vi "CAN Communication.vi"() -> ()   [LabVIEW 2011]
uses:
  <vilib>/Analysis/NI_AALBase.lvlib
panel:
  out "flag":bool
  out "Bias":dbl[](array[numeric]) format="%#.0f"
  out "ForceTorque":dbl[](array[numeric])
  in  "Overall TAP":enum32{"Graph", "CAN Activate"}(tab)
  in  "UNBIAS(SW)":bool
  in  "Control Box":T1={"Rotate & Translate"=FALSE, "rotation angle"=0.0, "Force Divider"=50.0, "Torque Divider"=2000.0}
  in  "BIAS(SW)":bool
  out "Tz":dbl(graph)
  out "Ty":dbl(graph)
  out "Tx":dbl(graph)
  out "Fz":dbl(graph)
  out "Fy":dbl(graph)
  out "Fx":dbl(graph)
  in  "Stop":bool
  in  "FT 출력":bool
  in  "Command":bool
  in  "Command":u16(ring)=11 items=["Not yet - Read Model Name", "Not yet - Read S/N", "Not yet - Read Firmware Ver.", "Set Communication ID", "Not yet - Read Communication ID", "UART version only - Set Baud-rate", "UART version only - Read Baud-rate", "Set Filter", "Not yet - Read Filter Setting", "F/T 1 sample Output", "F/T Output", "F/T Output Stop", "Reserved", "Reserved", "Set Output Rate", "Not yet -Read Output Rate", "Not yet -Bias Setting", "Not yet -Read Overload log"]
  in  "Set 2":T2={"Filter Type"=0, "Baud-rate"=0, "Output Rate"=0, "Cutoff Frequency"=0, "Receiving ID"=100, "Transmitting ID First "=1, "Transmitting ID Second"=2} {"Cutoff Frequency" items=["No filtering", "500Hz", "300Hz", "200Hz", "150Hz", "100Hz", "50Hz", "40Hz", "30Hz", "20Hz", "10Hz", "5Hz", "3Hz"]; "Output Rate" items=["200Hz", "10Hz", "20Hz", "50Hz", "100Hz", "200Hz", "333Hz", "500Hz", "1000Hz"]; "Baud-rate" items=["115,200", "921,600", "460,800", "230,400", "115,200", "57,600"]; "Filter Type" items=["None", "LowPass Filter"]}
  in  "Clear":bool
  in  "Auto Scale":bool
  in  "Torque Range":dbl(slide)=200.0 scale=0.0..10.0
  in  "Force Range":i32(slide)=200 scale=0.0..500.0
  out "CAN controller is started":bool
  out "Channel is active":bool
  in  "CAN Baudrate":u16(ring)=5120 items=["10 kBd"=7217, "20 kBd"=7192, "50 kBd"=7177, "100 kBd"=7172, "125 kBd "=7171, "250 kBd"=7169, "500 kBd"=7168, "800 kBd"=5632, "1000 kBd "=5120]
  in  "CAN Number":u32(ring) items=["CAN 0", "CAN 1"]
  out "Unbiased DATA":dbl[](array[numeric])
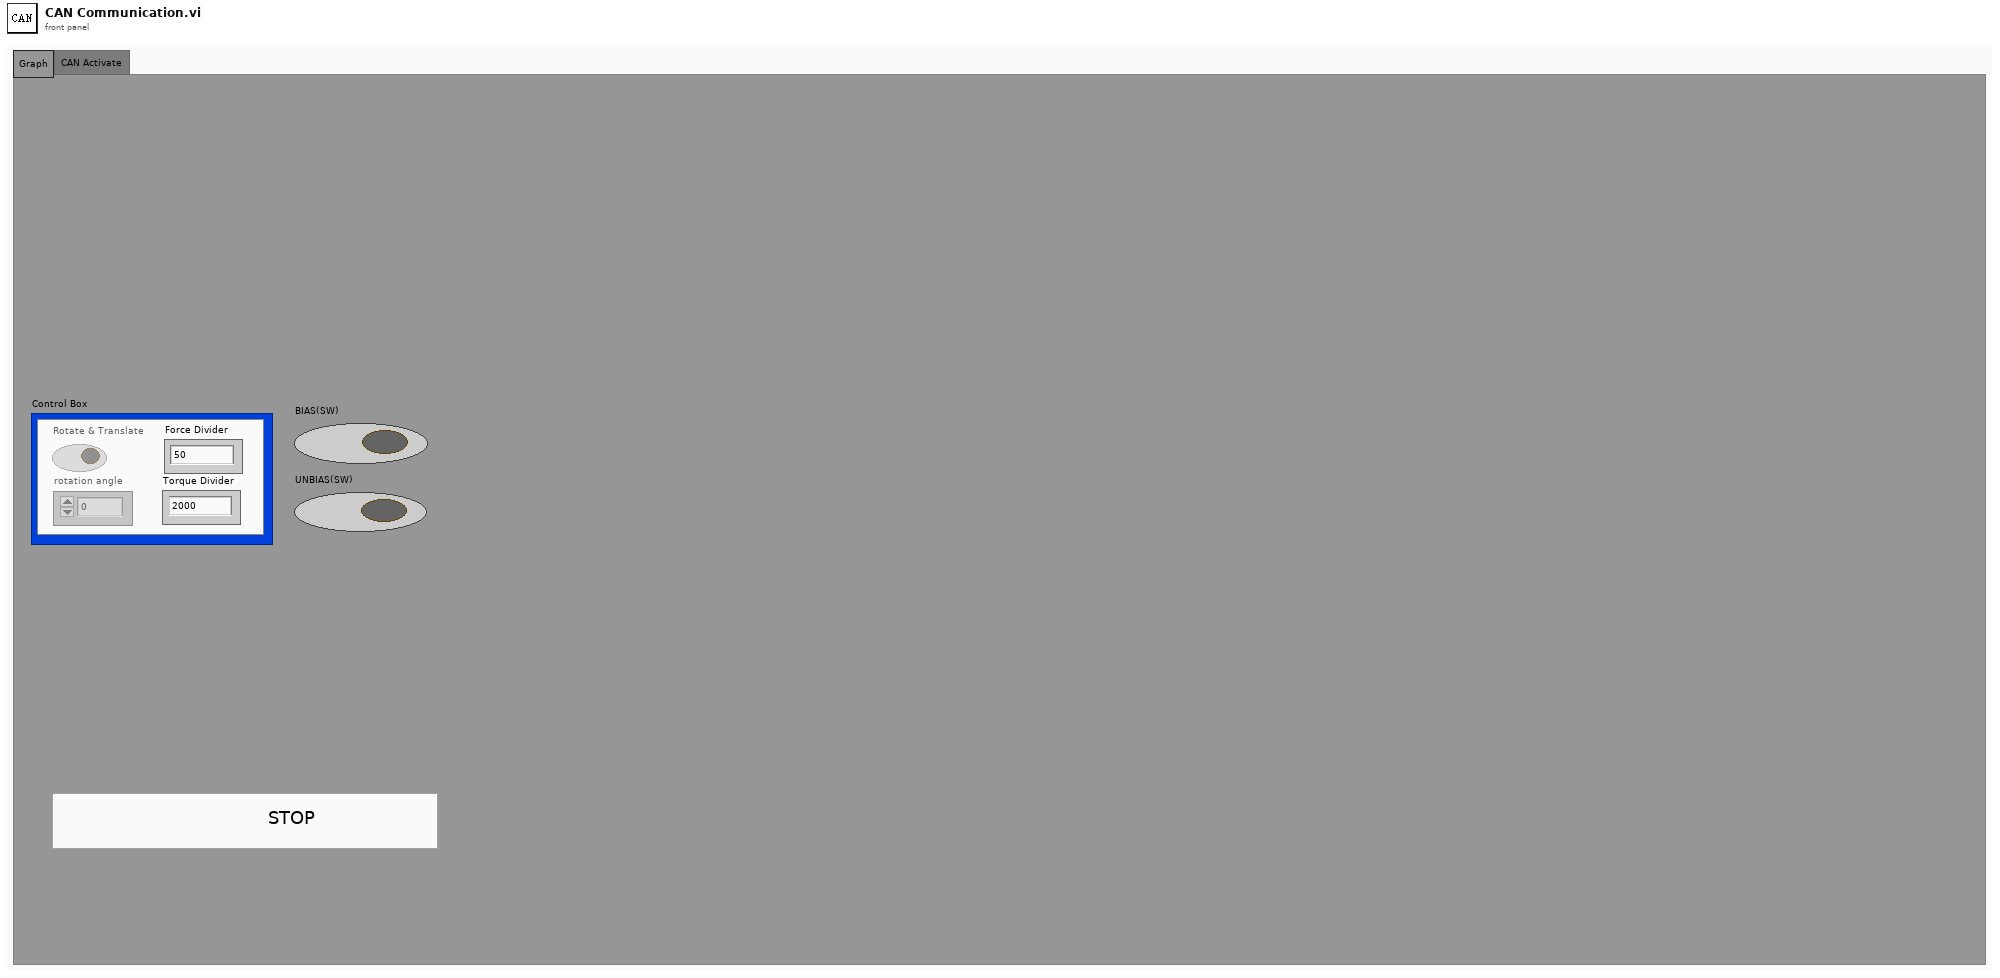
[diagram p1: front panel]
types:
  T1 = cluster{"Rotate & Translate":bool, "rotation angle":dbl, "Force Divider":dbl, "Torque Divider":dbl}
  T2 = cluster{"Filter Type":u16, "Baud-rate":u16, "Output Rate":u16, "Cutoff Frequency":u8, "Receiving ID":u8, "Transmitting ID First ":u8, "Transmitting ID Second":u8}
  T3 = cluster{"[0]":u8, "[1]":u8, "[2]":u8, "[3]":u8, "[4]":u8, "[5]":u8, "[6]":u8, "[7]":u8}[]
  T4 = cluster{"ForceTorque[0]":dbl, "ForceTorque[1]":dbl, "ForceTorque[2]":dbl, "ForceTorque[3]":dbl, "ForceTorque[4]":dbl, "ForceTorque[5]":dbl}
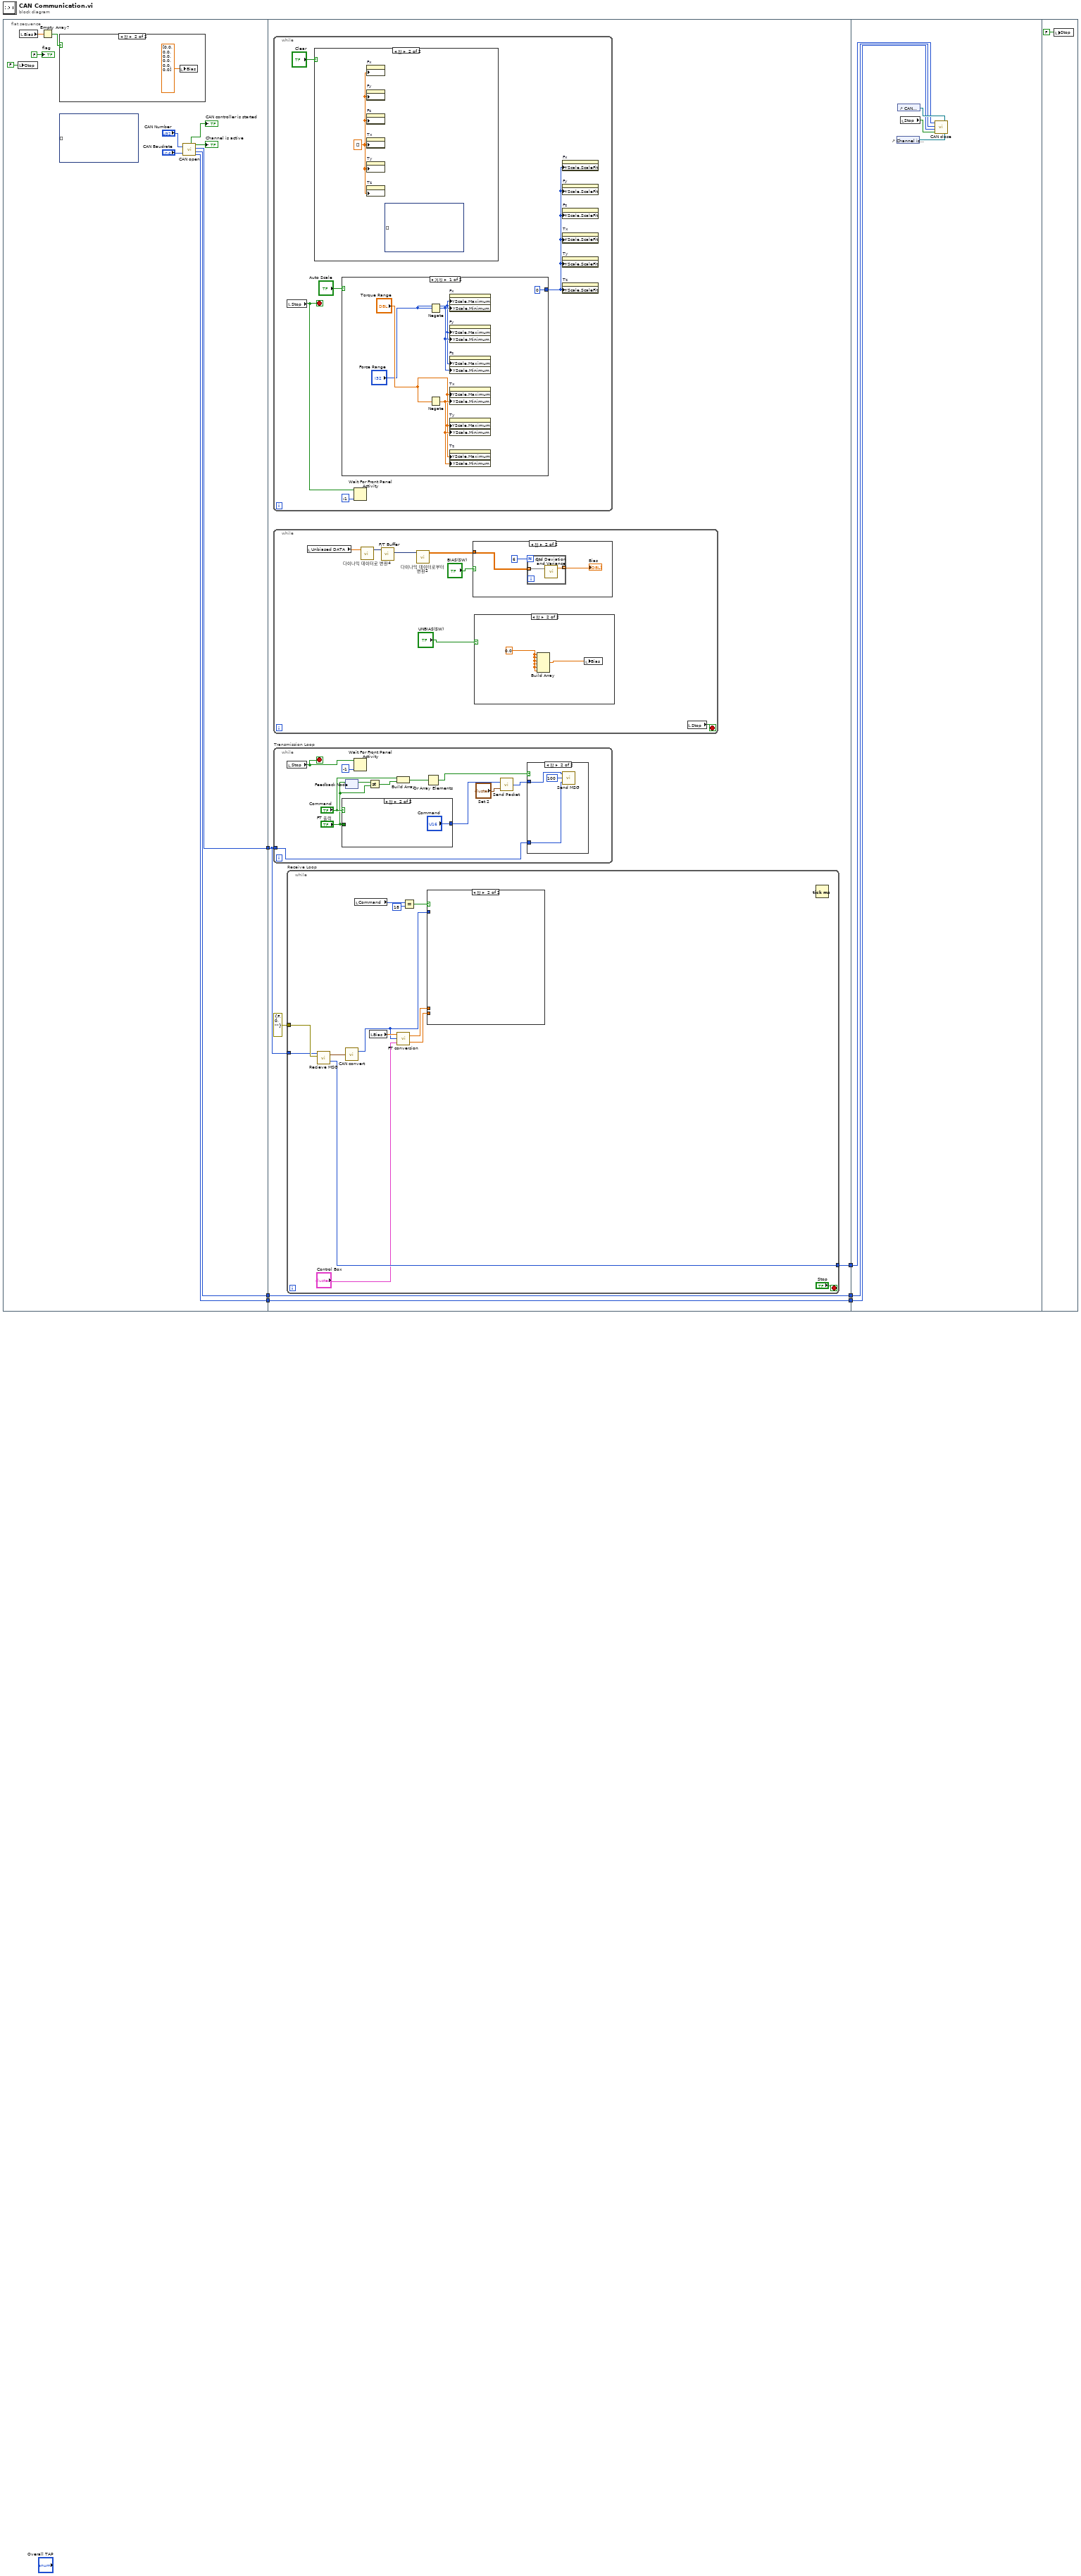
[diagram p0: block diagram]
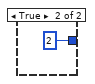
[diagram p3: hidden frame]
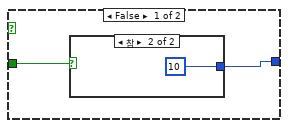
[diagram p7: hidden frame]
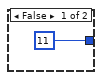
[diagram p8: hidden frame]
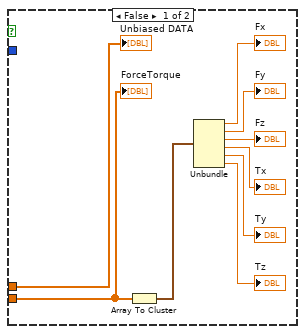
[diagram p10: hidden frame]
diagram:
  n1 = flat-sequence {
    tunnel: [w13] -> w6
    tunnel: [w12] -> w3
    tunnel: [w11] -> w2
    tunnel: w6 -> [w19]
    tunnel: [w22] -> w5
    tunnel: [w21] -> w4
    tunnel: w3 -> [w21]
    tunnel: w2 -> [w20]
    tunnel: [w20] -> w1
    tunnel: w5 -> [w95]
    tunnel: w4 -> [w93]
    tunnel: w1 -> [w92]
    frame #0 {
      (unwired) dynamicdata[] [] ("히스토리 데이터")
      n2 = local write "Stop"(FALSE ("정지 버튼")) -> ()
      n3 = local read "Bias"() -> (w10:dbl[])
      n4 = Empty Array?(array=w10) -> (empty?=w9:bool)
      n5 = case shown="참" w9 {
        frame False {
        }
        frame True {
          n6 = local write "Bias"(dbl[] [0.0, 0.0, 0.0, 0.0, 0.0, 0.0] ("Bias")) -> ()
        }
      }
      n7 = call "CAN open.vi"("CAN Baudrate"="CAN Baudrate", "CAN Number"="CAN Number") -> ("CAN Control Handle"=w11:u32, "Device Handle"=w12:u32, "CAN Channel Handle"=w13:u32, "Channel is active"=→"Channel is active":bool, "CAN controller is started"=→"CAN controller is started":bool)
      "flag" <- FALSE ("flag")
    }
    frame #1 {
      n8 = while {
        stop <- w27 stop-if-true
        n9 = local read "Stop"() -> (w27:bool)
        n10 = case shown="참" "Clear" {
          frame False {
          }
          frame True {
            w35 = dbl[] [] ("히스토리 데이터")
            (unwired) dynamicdata[] [] ("히스토리 데이터")
            n11 = property on="Fx" class="WFChart (엄격한)"("History Data"=w35) -> ()  [unwired: 2 in, 2 out]
            n12 = property on="Fy" class="WFChart (엄격한)"("History Data"=w35) -> ()  [unwired: 2 in, 2 out]
            n13 = property on="Fz" class="WFChart (엄격한)"("History Data"=w35) -> ()  [unwired: 2 in, 2 out]
            n14 = property on="Tx" class="WFChart (엄격한)"("History Data"=w35) -> ()  [unwired: 2 in, 2 out]
            n15 = property on="Ty" class="WFChart (엄격한)"("History Data"=w35) -> ()  [unwired: 2 in, 2 out]
            n16 = property on="Tz" class="WFChart (엄격한)"("History Data"=w35) -> ()  [unwired: 2 in, 2 out]
          }
        }
        n17 = case shown="거짓" "Auto Scale" {
          tunnel: [u8 0 ("Y 스케일.스케일 맞춤") u8 2 ("Y 스케일.스케일 맞춤")] -> w26
          frame False {
            n18 = Negate(x="Force Range") -> (-x=w32:i32)
            n19 = Negate(x="Torque Range") -> (-x=w33:dbl)
            n20 = property on="Fx" class="WFChart (엄격한)"("YScale.Maximum"="Force Range", "YScale.Minimum"=w32) -> ()  [unwired: 2 in, 2 out]
            n21 = property on="Fy" class="WFChart (엄격한)"("YScale.Maximum"="Force Range", "YScale.Minimum"=w32) -> ()  [unwired: 2 in, 2 out]
            n22 = property on="Fz" class="WFChart (엄격한)"("YScale.Maximum"="Force Range", "YScale.Minimum"=w32) -> ()  [unwired: 2 in, 2 out]
            n23 = property on="Tx" class="WFChart (엄격한)"("YScale.Maximum"="Torque Range", "YScale.Minimum"=w33) -> ()  [unwired: 2 in, 2 out]
            n24 = property on="Ty" class="WFChart (엄격한)"("YScale.Maximum"="Torque Range", "YScale.Minimum"=w33) -> ()  [unwired: 2 in, 2 out]
            n25 = property on="Tz" class="WFChart (엄격한)"("YScale.Maximum"="Torque Range", "YScale.Minimum"=w33) -> ()  [unwired: 2 in, 2 out]
          }
          frame True {
          }
        }
        n26 = Wait For Front Panel Activity(1:-1 ("timeout ms (-1 never timeout)"), 3:w27) -> ()  [unwired: 1 in, 1 out]
        n27 = property on="Fx" class="WFChart (엄격한)"("YScale.ScaleFit"=w26) -> ()  [unwired: 2 in, 2 out]
        n28 = property on="Fy" class="WFChart (엄격한)"("YScale.ScaleFit"=w26) -> ()  [unwired: 2 in, 2 out]
        n29 = property on="Fz" class="WFChart (엄격한)"("YScale.ScaleFit"=w26) -> ()  [unwired: 2 in, 2 out]
        n30 = property on="Tx" class="WFChart (엄격한)"("YScale.ScaleFit"=w26) -> ()  [unwired: 2 in, 2 out]
        n31 = property on="Ty" class="WFChart (엄격한)"("YScale.ScaleFit"=w26) -> ()  [unwired: 2 in, 2 out]
        n32 = property on="Tz" class="WFChart (엄격한)"("YScale.ScaleFit"=w26) -> ()  [unwired: 2 in, 2 out]
      }
      n33 = while {
        stop <- w42 stop-if-true
        n34 = local read "Unbiased DATA"() -> (w39:dbl[])
        n35 = call "다이나믹 데이터로 변환4"("Array"=w39) -> ("Dynamic Data Type"=w40:dynamicdata)  [unwired: 3 in]
        n36 = call "F/T Buffer"("Signals"=w40) -> ("Collected Signals"=w41:dynamicdata)  [unwired: 9 in, 1 out]
        n37 = call "다이나믹 데이터로부터 변환2"("Dynamic Data Type"=w41) -> ("Array"=w38:dbl[][])  [unwired: 3 in]
        n38 = case shown="참" "BIAS(SW)" {
          tunnel: w38 -> [_ w46]
          frame False {
          }
          frame True {
            n39 = for {
              N: 6 -> [_]
              tunnel: w46 -> [w49] mode=indexing
              tunnel: [w48] -> w45 mode=indexing
              n40 = call <vilib>:"Std Deviation and Variance.vi"("X"=w49) -> ("mean"=w48:dbl)  [unwired: 1 in, 2 out]
            }
            "Bias" <- w45
          }
        }
        n41 = case shown="참" "UNBIAS(SW)" {
          frame False {
          }
          frame True {
            w43 = 0.0
            n42 = Build Array(w43, w43, w43, w43, w43, w43) -> (w44:dbl[])
            n43 = local write "Bias"(w44) -> ()
          }
        }
        n44 = local read "Stop"() -> (w42:bool)
      }
      n45 = while "Transmission Loop" {
        tunnel: w19 -> [w59]
        stop <- w60 stop-if-true
        n46 = local read "Stop"() -> (w60:bool)
        n47 = case shown="참" "Command" {
          tunnel: [w62 "Command"] -> w53
          tunnel: "FT 출력" -> [w63 _]
          frame False {
            n48 = case shown="참" w63 {
              tunnel: [u16 11 ("Command") u16 10 ("Command")] -> w62
              frame False {
              }
              frame True {
              }
            }
          }
          frame True {
          }
        }
        n49 = feedback-in #1("FT 출력") -> ()
        n50 = feedback #1() -> (w57:bool)  [unwired: 1 in]
        n51 = Wait For Front Panel Activity(1:-1 ("timeout ms (-1 never timeout)"), 3:w60) -> ()  [unwired: 1 in, 1 out]
        n52 = Not Equal?(x=w57, y="FT 출력") -> (x != y?=w55:bool)
        n53 = Build Array("Command", w55) -> (w56:bool[])
        n54 = Or Array Elements(Boolean array=w56) -> (logical OR=w54:bool)
        n55 = call "Send Packet.vi"("Set"="Set 2", "Command"=w53) -> ("Packet"=w58:u8[])
        n56 = case shown="참" w54 {
          tunnel: w59 -> [_ w69]
          tunnel: w58 -> [_ w68]
          frame False {
          }
          frame True {
            n57 = call "Send MSG.vi"("CAN Channel Handle"=w69, "Arbitration ID"=u32 100, "Packet"=w68) -> ()
          }
        }
      }
      n58 = while "Receive Loop" {
        tunnel: w19 -> [w78]
        tunnel: errorcluster {"status"=FALSE, "code"=0, "source"=""} ("error in") -> [w82]
        tunnel: [w81] -> w22
        stop <- "Stop" stop-if-true
        n59 = call "Recieve MSG.vi"("error in"=w82, "CAN Channal Handle"=w78) -> ("CAN Channel Handle out"=w81:u32, "MSG  array"=w77:T3)  [unwired: 2 in]
        n60 = call "CAN convert.vi"("MSG  array"=w77) -> ("CAN"=w72:i32[])  [unwired: 1 out]
        n61 = local read "Command"() -> (w73:u16)
        n62 = local read "Bias"() -> (w79:dbl[])
        n63 = call "FT conversion.vi"("Control Box"="Control Box", "CAN"=w72, "Bias"=w79) -> ("ForceTorque"=w71:dbl[], "Unbiased DATA"=w74:dbl[])
        n64 = Equal?(x=w73, y=u16 18) -> (x = y?=w75:bool)
        n65 = case shown="참" w75 {
          tunnel: w72 -> [_ _]
          tunnel: w74 -> [w91 _]
          tunnel: w71 -> [w89 _]
          frame False {
            n66 = Array To Cluster(array=w89) -> (cluster=w90:T4)
            n67 = Unbundle(w90) -> ("ForceTorque[0]"=→"Fx":dbl, "ForceTorque[1]"=→"Fy":dbl, "ForceTorque[2]"=→"Fz":dbl, "ForceTorque[3]"=→"Tx":dbl, "ForceTorque[4]"=→"Ty":dbl, "ForceTorque[5]"=→"Tz":dbl)
            "Unbiased DATA" <- w91
            "ForceTorque" <- w89
          }
          frame True {
          }
        }
        n68 = Tick Count (ms)() -> ()  [unwired: 1 out]
      }
    }
    frame #2 {
      n69 = control-ref of="Channel is active"() -> (w97:refnum<vi>)
      n70 = control-ref of="CAN controller is started"() -> (w96:refnum<vi>)
      n71 = local read "Stop"() -> (w94:bool)
      n72 = call "CAN close.vi"("Channel is active"=w97, "CAN controller is started"=w96, "stop"=w94, "CAN Control Handle"=w92, "Device Handle"=w93, "CAN Channel Handle out"=w95) -> ()
    }
    frame #3 {
      n73 = local write "Stop"(FALSE ("정지 버튼")) -> ()
    }
  }
